vi "SCPI Read Program.vi"(1 "Cycles":u16, 2 "Steps":u16, 8 "error in (no error)":errorcluster, 11 "VISA resource name":refnum<visa-resource-name>) -> (0 "error out":errorcluster, 3 "VISA resource name out":refnum<visa-resource-name>)   [LabVIEW 2021, in "BK Precision 169XB.lvlib"]
doc: "Returns the actual voltage level and actual current level for a desired channel."
uses:
  BK Precision 169XB.lvlib
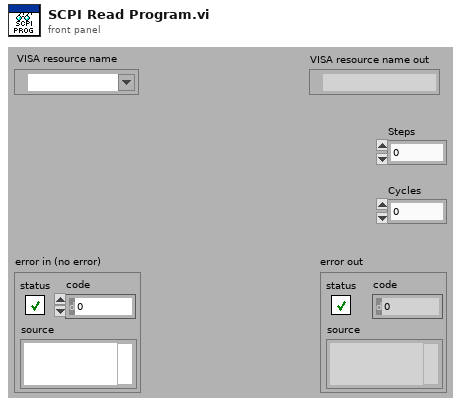
[diagram p1: front panel]
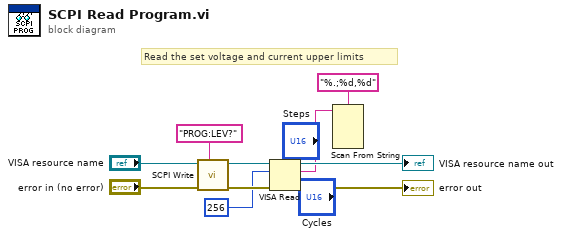
[diagram p0: block diagram]
diagram:
  # "Read the set voltage and current upper limits"
  n1 = call "SCPI Write.vi"("Input String"="PROG:LEV?", "error in (no error)"="error in (no error)", "VISA resource name"="VISA resource name") -> ("error out"=w8:errorcluster, "VISA resource name out"=w7:refnum<visa-resource-name>)  [unwired: 7 in]
  n2 = VISA Read(VISA resource name=w7, byte count=u32 256, error in (no error)=w8) -> (VISA resource name out=→"VISA resource name out":refnum<visa-resource-name>, read buffer=w3:string, error out=→"error out":errorcluster)  [unwired: 1 out]
  n3 = Scan From String(format string="%.;%d,%d", input string=w3) -> ()  [unwired: 6 in, 3 out]
